vi "Radio Get Peak.vi"(0 "a_data":dbl[](array[numeric]), 1 "a_startwav":dbl, 2 "a_endwav":dbl, 3 "a_Splinefactor":i16, 7 "error in (no error)":errorcluster) -> (16 "a_centroidnm out":dbl, 17 "a_centroidamp out":dbl, 18 "a_cwlnm out":dbl, 19 "a_cwlamp out":dbl, 20 "a_data out":dbl[](array[numeric]), 21 "function return":i16, 24 "a_peaknm out":dbl, 25 "a_peakamp out":dbl, 26 "a_fwhm out":dbl, 27 "error out":errorcluster)   [LabVIEW 2013, in "AVSirrad.lvlib"]
doc: "DLL_API short int __stdcall Radio_GetPeak\n(\n DataType *a_data,\n double a_startwav,\n double a_endwav,\n short int a_Splinefactor,\n double *a_peaknm,\n double *a_peakamp,\n double *a_fwhm,\n double *a_cwlnm,\n double *a_cwlamp,\n double *a_centroidnm,\n double *a_centroidamp\n);"
uses:
  AVSirrad.lvlib
  AVSIRRAD/Examples/Labview/build/AVSirrad.dll
panel:
  in  "a_centroidamp":dbl
  in  "a_centroidnm":dbl
  in  "a_cwlamp":dbl
  in  "a_cwlnm":dbl
  in  "a_fwhm":dbl
  in  "a_peakamp":dbl
  in  "a_peaknm":dbl
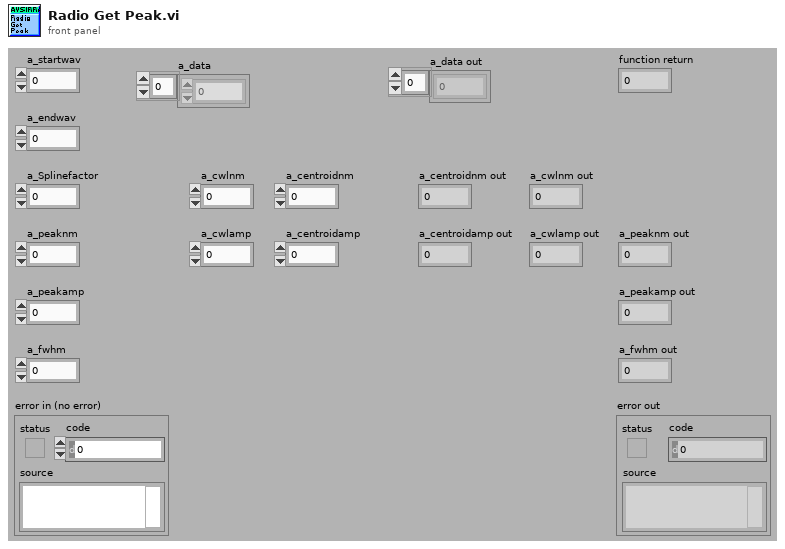
[diagram p1: front panel]
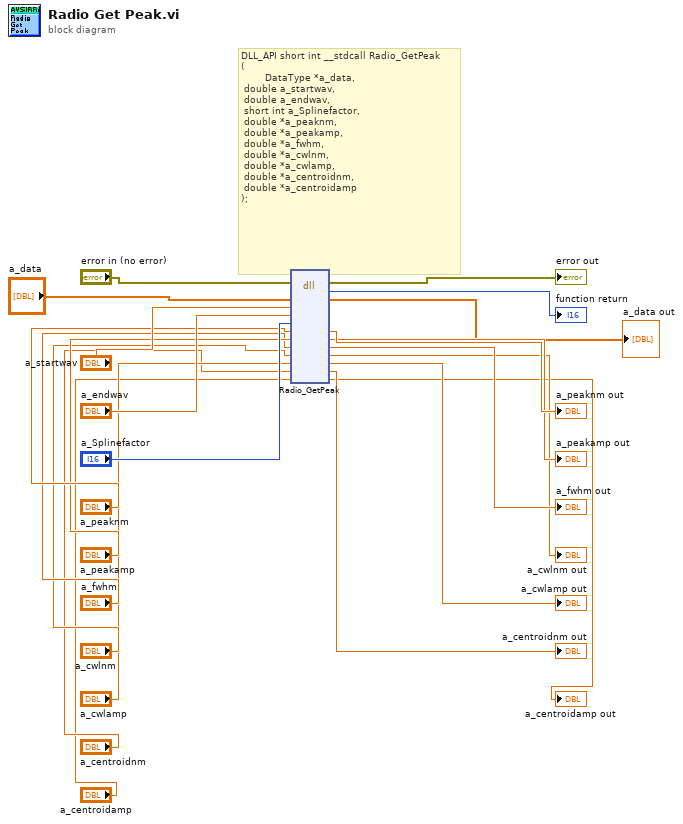
[diagram p0: block diagram]
diagram:
  # "DLL_API short int __stdcall Radio_GetPeak\n(\n        DataType *a_data,\n\tdouble a_startwav,\n\tdouble a_endwav,\n\tshort int a_Splinefactor,\n\tdouble *a_peaknm,\n\tdouble *a_peakamp,\n\tdouble *a_fwhm,\n\tdouble *a_cwlnm,\n\tdouble *a_cwlamp,\n\tdouble *a_centroidnm,\n\tdouble *a_centroidamp\n);"
  n1 = dll-call lib="C:/AVSIRRAD/Examples/Labview/build/AVSirrad.*" fn="Radio_GetPeak"(error in="error in (no error)", "a_data"="a_data", "a_startwav"="a_startwav", "a_endwav"="a_endwav", "a_Splinefactor"="a_Splinefactor", "a_peaknm"="a_peaknm", "a_peakamp"="a_peakamp", "a_fwhm"="a_fwhm", "a_cwlnm"="a_cwlnm", "a_cwlamp"="a_cwlamp", "a_centroidnm"="a_centroidnm", "a_centroidamp"="a_centroidamp") -> (error out=→"error out":errorcluster, "return type"=→"function return":i16, "a_data"=→"a_data out":dbl[], "a_peaknm"=→"a_peaknm out":dbl, "a_peakamp"=→"a_peakamp out":dbl, "a_fwhm"=→"a_fwhm out":dbl, "a_cwlnm"=→"a_cwlnm out":dbl, "a_cwlamp"=→"a_cwlamp out":dbl, "a_centroidnm"=→"a_centroidnm out":dbl, "a_centroidamp"=→"a_centroidamp out":dbl)  [unwired: 5 in, 1 out]
